vi "PFI-28000-Card-28144_Set Fault Check Interval.vi"(8 "error in (no error)":errorcluster, 10 "Fault Check Interval":i32, 11 "PFI-28000-Card-28144 in":refnum<class "PFI-28000-Card-28144.lvclass">) -> (0 "error out":errorcluster, 3 "PFI-28000-Card-28144 out":refnum<class "PFI-28000-Card-28144.lvclass">)   [LabVIEW 2017, in "PFI-28000-Card-28144.lvclass"]
uses:
  PFI-28000-Card-28144.lvclass
  C:/wc/07143 Precision Filters 28000 Support/Driver/source/Card/PFI-28000-Card.lvclass
  Channel/PFI-28000-Channel.lvclass
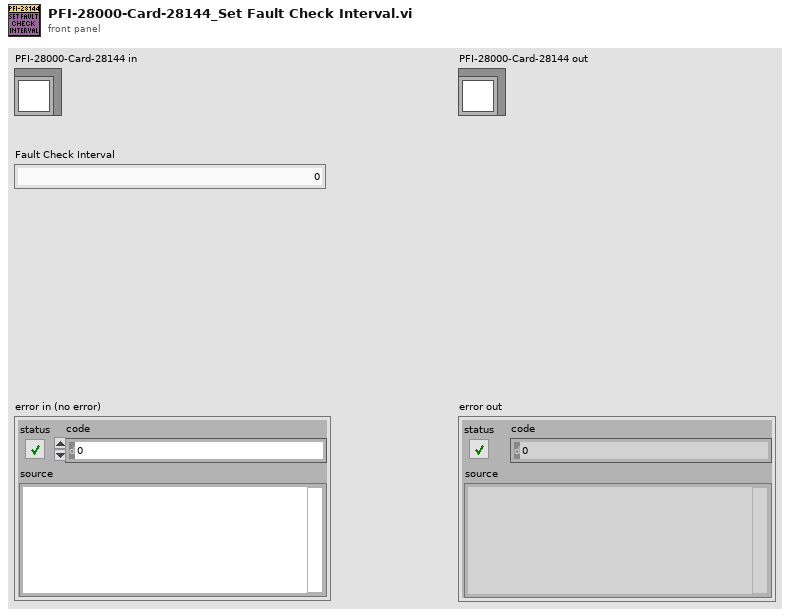
[diagram p1: front panel]
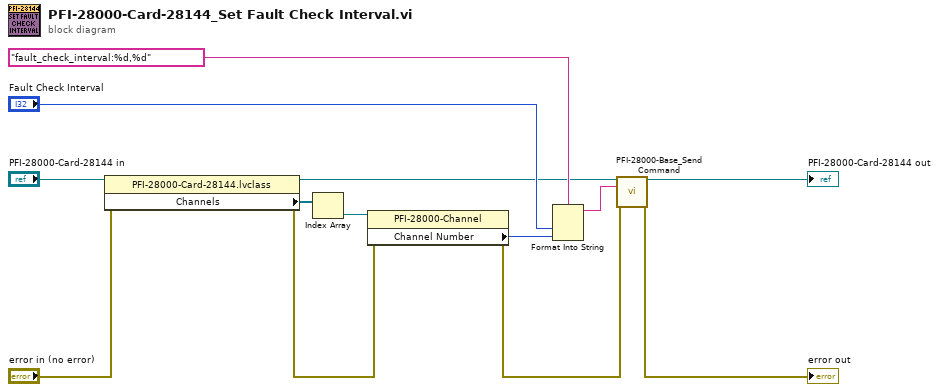
[diagram p0: block diagram]
diagram:
  n1 = property class="PFI-28000-Card-28144.lvclass"(reference="PFI-28000-Card-28144 in", error in="error in (no error)") -> (reference out=w5:refnum<class "PFI-28000-Card-28144.lvclass">, error out=w10:errorcluster, "Channels"=w9:refnum<class "PFI-28000-Channel.lvclass">[])
  n2 = Index Array(array=w9) -> (element=w8:refnum<class "PFI-28000-Channel.lvclass">)  [unwired: 1 in]
  n3 = property class="PFI-28000-Channel"(reference=w8, error in=w10) -> (error out=w2:errorcluster, "Channel Number"=w7:i32)  [unwired: 1 out]
  n4 = Format Into String(format string="fault_check_interval:%d,%d" ("empty string"), "Fault Check Interval", w7) -> (resulting string=w3:string)  [unwired: 2 in, 1 out]
  n5 = call-dynamic "PFI-28000-Base_Send Command.vi"("PFI-28000-Base in"=w5, "Command"=w3, "error in (no error)"=w2) -> ("PFI-28000-Base out"=→"PFI-28000-Card-28144 out":refnum<class "PFI-28000-Card-28144.lvclass">, "error out"=→"error out":errorcluster)  [unwired: 11 in]
